vi "Read.vi"(8 "error in (no error)":errorcluster, 10 "byte count":u32=1 format="%x", 11 "MODBUS in":refnum<class "PL Modbus Client.lvclass">) -> (0 "error out":errorcluster, 2 "read buffer":string, 3 "MODBUS out":refnum<class "PL Modbus Client.lvclass">)   [LabVIEW 2015, in "PL Modbus Client.lvclass"]
doc: "Reads bytes from specified interface."
uses:
  PL Modbus Client.lvclass
  PL Modbus Client.lvclass/PL Modbus Client.ctl
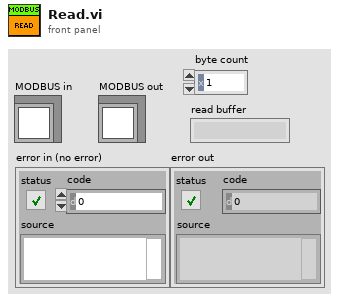
[diagram p1: front panel]
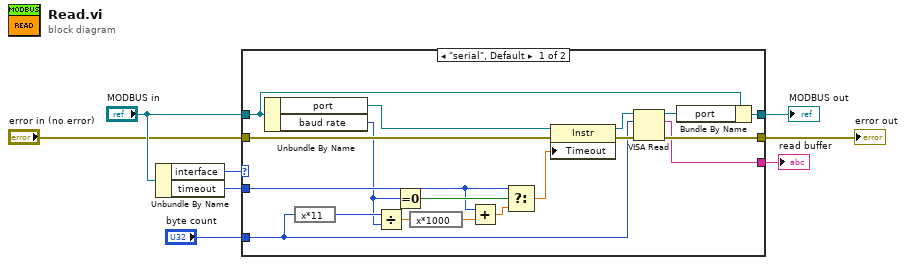
[diagram p0: block diagram]
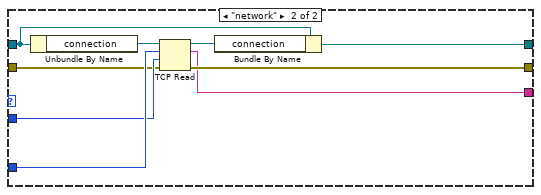
[diagram p2: hidden frame]
diagram:
  n1 = Unbundle By Name("MODBUS in") -> ("interface"=w8:enum16{"serial", "network"}, "timeout"=w6:u32)
  n2 = case shown="\"serial\", Default" w8 {
    tunnel: "MODBUS in" -> [w26 w35]
    tunnel: w6 -> [w13 w31]
    tunnel: "error in (no error)" -> [w10 w30]
    tunnel: [w24 w34] -> w4
    tunnel: [w23 w29] -> w3
    tunnel: [w22 w27] -> w2
    tunnel: "byte count" -> [w18 w32]
    frame "serial", Default {
      n3 = Unbundle By Name(w26) -> ("port"=w11:refnum<visa-resource-name>, "baud rate"=w9:u32)
      n4 = expression code="x*11"(w18) -> (w16:u32)
      n5 = Divide(x=w16, y=w9) -> (x/y=w15:dbl)
      n6 = Equal To 0?(x=w9) -> (x = 0?=w19:bool)
      n7 = expression code="x*1000"(w15) -> (w12:dbl)
      n8 = Add(x=w13, y=w12) -> (x+y=w14:dbl)
      n9 = Select(t=w13, s=w19, f=w14) -> (s? t:f=w17:dbl)
      n10 = property class="Instr"(reference=w11, error in=w10, "Timeout"=w17) -> (reference out=w20:refnum<visa-resource-name>, error out=w21:errorcluster)
      n11 = VISA Read(VISA resource name=w20, byte count=w18, error in (no error)=w21) -> (VISA resource name out=w25:refnum<visa-resource-name>, read buffer=w22:string, error out=w23:errorcluster)  [unwired: 1 out]
      n12 = Bundle By Name(cluster=w26, "port"=w25) -> (w24:refnum<class "PL Modbus Client.lvclass">)
    }
    frame "network" {
      n13 = Unbundle By Name(w35) -> ("connection"=w33:refnum<k5>)
      n14 = TCP Read(connection ID=w33, bytes to read=w32, error in (no error)=w30, 9:w31) -> (connection ID out=w28:refnum<k5>, data out=w27:string, error out=w29:errorcluster)  [unwired: 1 in]
      n15 = Bundle By Name(cluster=w35, "connection"=w28) -> (w34:refnum<class "PL Modbus Client.lvclass">)
    }
  }
  "MODBUS out" <- w4
  "read buffer" <- w2
  "error out" <- w3
